vi "mod_Modulo Integrator (real array).vi"(6 "reset?":bool, 8 "initial y":dbl format="%.2f", 9 "modulo":dbl=-1.0 format="%.2f", 11 "x":dbl[](array[numeric]) format="%.2f") -> (3 "y":dbl[](array[numeric]) format="%.2f")   [LabVIEW 2020, in "niAMT.lvlib"]
uses:
  <vilib>/addons/Modulation/niAMT.lvlib
panel:
  # "H(z) = z/(z-1)"
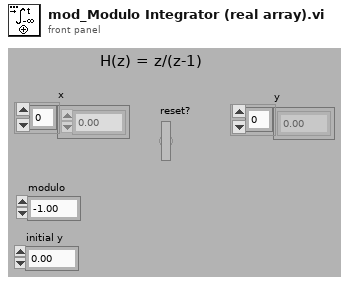
[diagram p1: front panel]
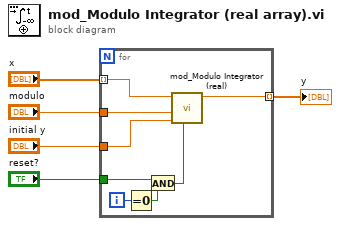
[diagram p0: block diagram]
diagram:
  n1 = for {
    tunnel: "x" -> [w13] mode=indexing
    tunnel: "modulo" -> [w6]
    tunnel: "initial y" -> [w12]
    tunnel: "reset?" -> [w9]
    tunnel: [w7] -> w1 mode=indexing
    i -> [w11]
    n2 = Equal To 0?(x=w11) -> (x = 0?=w10:bool)
    n3 = And(x=w9, y=w10) -> (x .and. y?=w8:bool)
    n4 = call <vilib>:"mod_Modulo Integrator (real).vi"("reset?"=w8, "initial y"=w12, "modulo"=w6, "x"=w13) -> ("y"=w7:dbl)  [unwired: 7 out]
  }
  "y" <- w1
